vi "CheckValidAction.vi"(9 "Starting Game Piece":T1, 10 "y":i32, 11 "x":i32) -> (3 "Boolean":bool)   [LabVIEW 2018]
uses:
  Piece.ctl
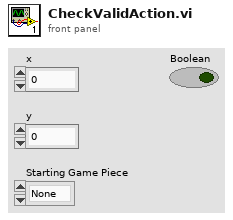
[diagram p1: front panel]
types:
  T1 = typedef "Piece.ctl" = enum16{"None", "Cargo", "Hatch Panel"}
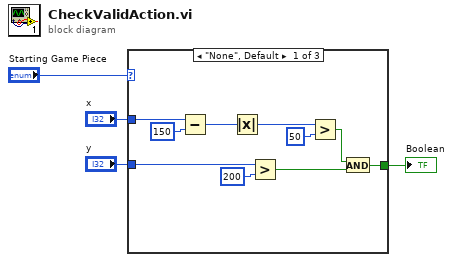
[diagram p0: block diagram]
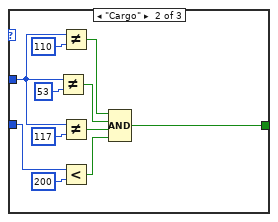
[diagram p2: hidden frame]
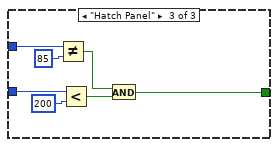
[diagram p3: hidden frame]
diagram:
  n1 = case shown="\"None\", Default" "Starting Game Piece" {
    tunnel: "x" -> [w13 w20 w32]
    tunnel: "y" -> [w14 w25 w28]
    tunnel: [w5 w15 w29] -> w3
    frame "None", Default {
      n2 = Subtract(x=w13, y=150) -> (x-y=w9:i32)
      n3 = Absolute Value(x=w9) -> (abs(x)=w10:i32)
      n4 = Greater?(x=w14, y=200) -> (0:w12:bool)
      n5 = Greater?(x=w10, y=50) -> (0:w11:bool)
      n6 = And(x=w11, y=w12) -> (x .and. y?=w5:bool)
    }
    frame "Cargo" {
      n7 = Not Equal?(x=w20, y=53) -> (x != y?=w18:bool)
      n8 = Not Equal?(x=w20, y=110) -> (x != y?=w19:bool)
      n9 = Not Equal?(x=w20, y=117) -> (x != y?=w17:bool)
      n10 = Less?(x=w25, y=200) -> (x < y?=w16:bool)
      n11 = Compound Arithmetic op=AND(w19, w18, w17, w16) -> (w15:bool)
    }
    frame "Hatch Panel" {
      n12 = Not Equal?(x=w32, y=85) -> (x != y?=w30:bool)
      n13 = Less?(x=w28, y=200) -> (x < y?=w27:bool)
      n14 = And(x=w30, y=w27) -> (x .and. y?=w29:bool)
    }
  }
  "Boolean" <- w3
